vi "StopAcquisitionRequestRoutedMessage_Send.vi"(8 "error in (no error)":errorcluster, 10 "StopAcquisitionRequest":T1, 11 "Qbus in":refnum<class "Qbus.lvclass">) -> (0 "error out":errorcluster, 3 "Qbus out":refnum<class "Qbus.lvclass">)   [LabVIEW 2017, in "CmsAcquisition.lvlib"]
uses:
  <vilib>/addons/InsightCM/Devices/Shared/Cms/CmsAcquisition/CmsAcquisition.lvlib
  <vilib>/addons/Qbus/Qbus.lvclass
  <vilib>/addons/InsightCM/Devices/Shared/Cms/CmsAcquisition/controls/StopAcquisitionRequest.ctl
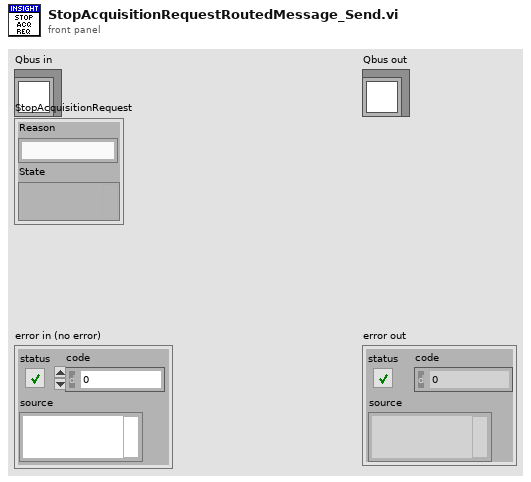
[diagram p1: front panel]
types:
  T1 = typedef "CmsAcquisition.lvlib/StopAcquisitionRequest.ctl" = cluster{"Reason":string, "State":variant}
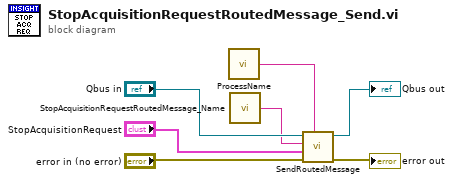
[diagram p0: block diagram]
diagram:
  n1 = call <vilib>:"ProcessName.vi"() -> ("process name"=w1:string)  [unwired: 5 in]
  n2 = call <vilib>:"StopAcquisitionRequestRoutedMessage_Name.vi"() -> ("message name"=w2:string)  [unwired: 5 in]
  n3 = call <vilib>:"SendRoutedMessage.vi"("listener process"=w1, "error in (no error)"="error in (no error)", "message value"="StopAcquisitionRequest", "message name"=w2, "Qbus in"="Qbus in") -> ("error in (no error)"=→"error out":errorcluster, "Qbus out"=→"Qbus out":refnum<class "Qbus.lvclass">)  [unwired: 5 in]
